vi "Request Motors with Encoders State.vi"(8 "error in (no error)":errorcluster, 9 "Requestor Queue":refnum<class "Message Enqueuer.lvclass">, 10 "Current State Msg":refnum<class "Current State Msg.lvclass">, 11 "Comp Motors with Encoders in":refnum<class "Comp Motors with Encoders.lvclass">) -> (0 "error out":errorcluster, 3 "Comp Motors with Encoders out":refnum<class "Comp Motors with Encoders.lvclass">)   [LabVIEW 2014, in "Comp Motors with Encoders.lvlib" / "Comp Motors with Encoders.lvclass"]
uses:
  Comp Motors with Encoders.lvclass
  Robot/Motor with Encoders/Motors with Encoders Messages/Current State Msg/Current State Msg.lvclass
  <vilib>/ActorFramework/Message Enqueuer/Message Enqueuer.lvclass
  Robot/Motor with Encoders/Motors with Encoders Class/Motors with Encoders.lvclass
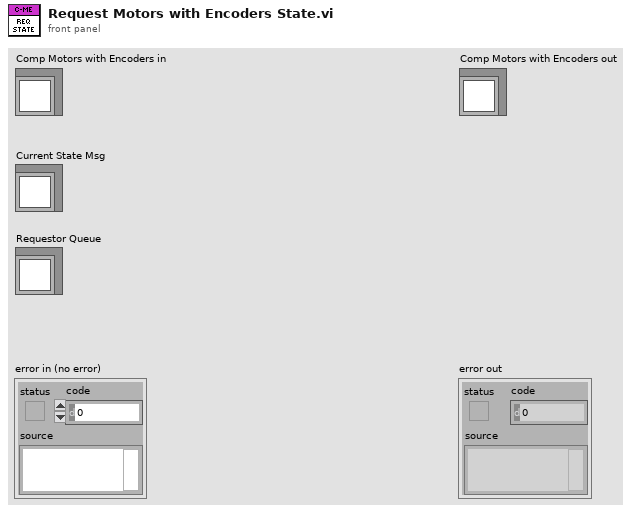
[diagram p1: front panel]
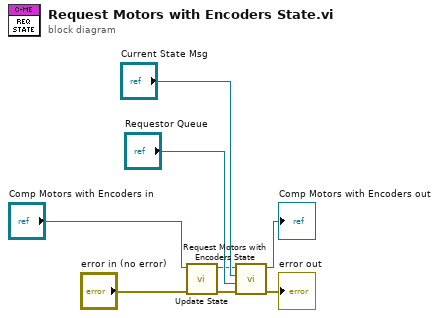
[diagram p0: block diagram]
diagram:
  n1 = call-dynamic "Update State.vi"("error in (no error)"="error in (no error)", "Comp Motors with Encoders in"="Comp Motors with Encoders in") -> ("error out"=w1:errorcluster, "Comp Motors with Encoders out"=w2:refnum<class "Comp Motors with Encoders.lvclass">)  [unwired: 8 in]
  n2 = call-parent "Request Motors with Encoders State.vi"("error in (no error)"=w1, "Requestor Queue"="Requestor Queue", "Current State Msg"="Current State Msg", "Motors with Encoders in"=w2) -> ("error out"=→"error out":errorcluster, "Motors with Encoders out"=→"Comp Motors with Encoders out":refnum<class "Comp Motors with Encoders.lvclass">)  [unwired: 6 in]
